vi "Usage3.vi"() -> ()   [LabVIEW 2017]
uses:
  SLSC Switch Consumer/SLSC Switch Consumer.lvclass
  C:/github/niveristand-slsc-switch-message-library/Includes/CDMessaging.lvlibp/Consumer/Abstract Consumer/Abstract Consumer.lvclass
  Includes/CDMessaging.lvlibp/Switch/Abstract Switch Init Parameters/Abstract Switch Init Parameters.lvclass
  C:/github/niveristand-slsc-switch-message-library/Includes/CDMessaging.lvlibp/Parameters/Abstract Init Parameters/Abstract Init Parameters.lvclass
  Includes/CDMessaging.lvlibp/Consumer/Abstract Consumer/Abstract Consumer.lvclass
  Includes/CDMessaging.lvlibp/Producer/Abstract Producer/Abstract Producer.lvclass
  Includes/CDMessaging.lvlibp/Message Queue/Message Queue/Message Queue.lvclass
  C:/github/niveristand-slsc-switch-message-library/Includes/CDMessaging.lvlibp/Message Queue/Abstract Message Queue/Abstract Message Queue.lvclass
  Includes/CDMessaging.lvlibp/Parameters/Abstract Init Parameters/Abstract Init Parameters.lvclass
  Includes/CDMessaging.lvlibp/Switch/Switch Connect Message/Switch Connect Message.lvclass
  C:/github/niveristand-slsc-switch-message-library/Includes/CDMessaging.lvlibp/Message/Abstract Message/Abstract Message.lvclass
  Includes/CDMessaging.lvlibp/Switch/Switch Disconnect Message/Switch Disconnect Message.lvclass
  Includes/CDMessaging.lvlibp/Switch/Switch Disconnect All Message/Switch Disconnect All Message.lvclass
  Includes/CDMessaging.lvlibp/Message/Shutdown Message/Shutdown Message.lvclass
panel:
  in  "Disconnect":bool
  in  "Disconnect All":bool
  in  "Connect":bool
  in  "Shutdown":bool
  out "error out":errorcluster
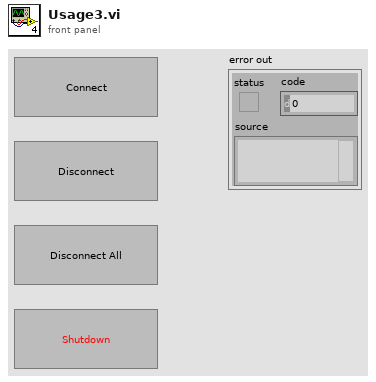
[diagram p1: front panel]
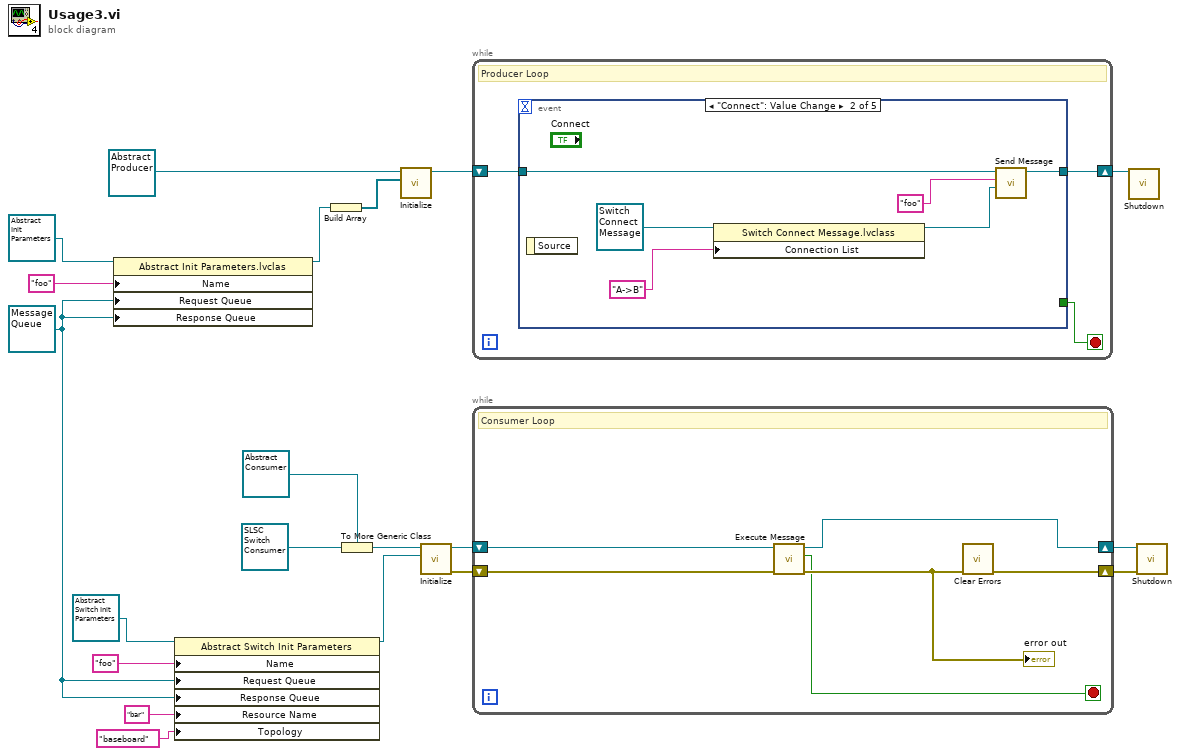
[diagram p0: block diagram]
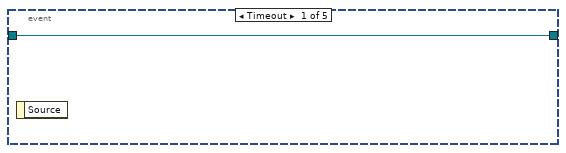
[diagram p2: hidden frame]
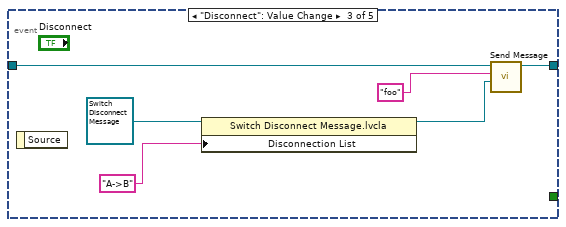
[diagram p3: hidden frame]
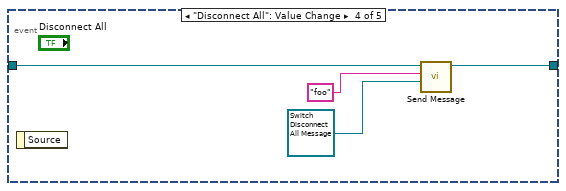
[diagram p4: hidden frame]
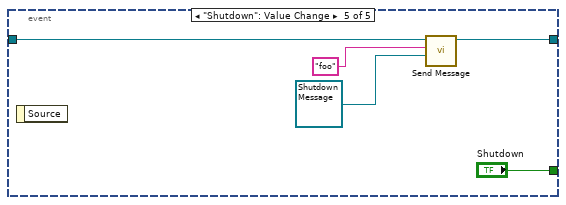
[diagram p5: hidden frame]
diagram:
  w1 = refnum<class "Message Queue.lvclass"> refnum ("Message Queue Library.lvlib:Message Queue.lvclass")
  n1 = property class="Abstract Init Parameters.lvclas"(reference=refnum<class "Abstract Init Parameters.lvclass"> refnum ("Message Queue Library.lvlib:Abstract Init Parameters.lvclass"), "Name"="foo", "Request Queue"=w1, "Response Queue"=w1) -> (reference out=w4:refnum<class "Abstract Init Parameters.lvclass">)  [unwired: 1 in, 1 out]
  n2 = property class="Abstract Switch Init Parameters"(reference=refnum<class "Abstract Switch Init Parameters.lvclass"> refnum ("Message Queue Library.lvlib:Abstract Switch Init Parameters.lvclass"), "Name"="foo", "Request Queue"=w1, "Response Queue"=w1, "Resource Name"="bar", "Topology"="baseboard") -> (reference out=w17:refnum<class "Abstract Switch Init Parameters.lvclass">)  [unwired: 1 in, 1 out]
  n3 = Build Array(w4) -> (w7:refnum<class "Abstract Init Parameters.lvclass">[])
  n4 = To More Generic Class(target class=refnum<class "Abstract Consumer.lvclass"> refnum ("Abstract Consumer in"), reference=refnum<class "SLSC Switch Consumer.lvclass"> refnum ("Message Queue Library.lvlib:SLSC Switch Consumer.lvclass")) -> (generic class reference=w9:refnum<class "Abstract Consumer.lvclass">)
  n5 = call "Initialize.vi"("Parameters in"=w7, "Abstract Producer in"=refnum<class "Abstract Producer.lvclass"> refnum ("Message Queue Library.lvlib:Abstract Producer.lvclass")) -> ("Abstract Producer out"=w3:refnum<class "Abstract Producer.lvclass">)  [unwired: 8 in, 1 out]
  n6 = call "Initialize.vi"("Parameters in"=w17, "Abstract Consumer in"=w9) -> ("error out"=w20:errorcluster, "Abstract Consumer out"=w16:refnum<class "Abstract Consumer.lvclass">)  [unwired: 8 in]
  n7 = while {
    shift-right: [w21] -> w2
    shift-left: w3 -> [w22]
    stop <- w23 stop-if-true
    # "Producer Loop"
    n8 = event shown="[1] \"Connect\": Value Change" {
      selector: _ -> [_ _ _ _ _]
      dyn-events: _ -> [_ _ _ _ _]
      timeout: _ -> [_ _ _ _ _]
      tunnel: [_ _ _ _ "Shutdown"] -> w23
      tunnel: w22 -> [w24 w28 w33 w39 w43]
      tunnel: [w24 w25 w31 w37 w41] -> w21
      event Timeout {
        n9 = event-data() -> ()  [unwired: 1 in, 1 out]
      }
      event "Connect": Value Change {
        n10 = event-data() -> ()  [unwired: 1 in, 1 out]
        n11 = property class="Switch Connect Message.lvclass"(reference=refnum<class "Switch Connect Message.lvclass"> refnum ("Message Queue Library.lvlib:Switch Connect Message.lvclass"), "Connection List"="A->B") -> (reference out=w27:refnum<class "Switch Connect Message.lvclass">)  [unwired: 1 in, 1 out]
        n12 = call-dynamic "Send Message.vi"("Message in"=w27, "Consumer in"="foo" ("Name"), "Abstract Producer in"=w28) -> ("Abstract Producer out"=w25:refnum<class "Abstract Producer.lvclass">)  [unwired: 6 in, 2 out]
      }
      event "Disconnect": Value Change {
        n13 = event-data() -> ()  [unwired: 1 in, 1 out]
        n14 = property class="Switch Disconnect Message.lvcla"(reference=refnum<class "Switch Disconnect Message.lvclass"> refnum ("Message Queue Library.lvlib:Switch Disconnect Message.lvclass"), "Disconnection List"="A->B" ("Connection List")) -> (reference out=w32:refnum<class "Switch Disconnect Message.lvclass">)  [unwired: 1 in, 1 out]
        n15 = call-dynamic "Send Message.vi"("Message in"=w32, "Consumer in"="foo" ("Name"), "Abstract Producer in"=w33) -> ("Abstract Producer out"=w31:refnum<class "Abstract Producer.lvclass">)  [unwired: 6 in, 2 out]
      }
      event "Disconnect All": Value Change {
        n16 = event-data() -> ()  [unwired: 1 in, 1 out]
        n17 = call-dynamic "Send Message.vi"("Message in"=refnum<class "Switch Disconnect All Message.lvclass"> refnum ("Message Queue Library.lvlib:Switch Disconnect All Message.lvclass"), "Consumer in"="foo" ("Name"), "Abstract Producer in"=w39) -> ("Abstract Producer out"=w37:refnum<class "Abstract Producer.lvclass">)  [unwired: 6 in, 2 out]
      }
      event "Shutdown": Value Change {
        n18 = event-data() -> ()  [unwired: 1 in, 1 out]
        n19 = call-dynamic "Send Message.vi"("Message in"=refnum<class "Shutdown Message.lvclass"> refnum ("Message Queue Library.lvlib:Shutdown Message.lvclass"), "Consumer in"="foo" ("Name"), "Abstract Producer in"=w43) -> ("Abstract Producer out"=w41:refnum<class "Abstract Producer.lvclass">)  [unwired: 6 in, 2 out]
      }
    }
  }
  n20 = while {
    shift-right: [w46] -> w13
    shift-left: w20 -> [w51]
    shift-right: [w47] -> w12
    shift-left: w16 -> [w48]
    stop <- w49 stop-if-true
    # "Consumer Loop"
    n21 = call "Execute Message.vi"("error in (no error)"=w51, "Abstract Consumer in"=w48) -> ("error out"=w50:errorcluster, "Stop?"=w49:bool, "Abstract Consumer out"=w47:refnum<class "Abstract Consumer.lvclass">)  [unwired: 7 in]
    "error out" <- w50
    n22 = call <vilib>:"Clear Errors.vi"("error in (no error)"=w50) -> ("error out"=w46:errorcluster)  [unwired: 5 in, 1 out]
  }
  n23 = call "Shutdown.vi"("Abstract Producer in"=w2) -> ()  [unwired: 9 in, 2 out]
  n24 = call "Shutdown.vi"("error in (no error)"=w13, "Abstract Consumer in"=w12) -> ()  [unwired: 8 in, 2 out]
